vi "Process Collision.vi"(11 "Ball-Edge in":refnum<class "Ball-Edge.lvclass">) -> (3 "Ball-Edge out":refnum<class "Ball-Edge.lvclass">)   [LabVIEW 2021, in "Ball-Edge.lvclass"]
doc: "MIT Licence\nCopyright (c) 2024 David Grollier"
uses:
  Ball-Edge.lvclass
  C:/Users/David/Documents/GameSoccerSpace/Source/Collision/Collision.lvclass
  Collision type.ctl
  Game Componants/Game Board Component/Fixed/Board/Rectangle/Rectangle.lvclass
  Collision.lvclass/Collision.ctl
  Game Componants/Game Board Component/Movable/Movable.lvclass/Movable.ctl
  Game Componants/Game Board Component/Fixed/Board/Rectangle/Rectangle.lvclass/Rectangle.ctl
  Ball-Edge.lvclass/Ball-Edge.ctl
  Game Componants/Game Board Component/Movable/Movable.lvclass
  C:/Users/David/Documents/GameSoccerSpace/Source/Game Componants/Game Board Component/Game Board Component.lvclass
  Type Def/Coordinates.ctl
  Collision.lvclass
panel:
  out "sqrt(x)":dbl
  out "test type":T1
  out "test collision":bool
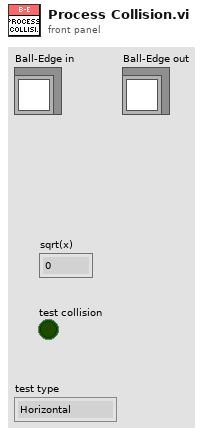
[diagram p1: front panel]
types:
  T1 = typedef "Ball-Edge.lvclass/Collision type.ctl" = enum16{"Horizontal", "Vertical", "Corner"}
  T2 = typedef "Coordinates.ctl" = cluster{"x":dbl, "y":dbl}
  T3 = cluster{"left":i16, "top":i16, "right":i16, "bottom":i16}
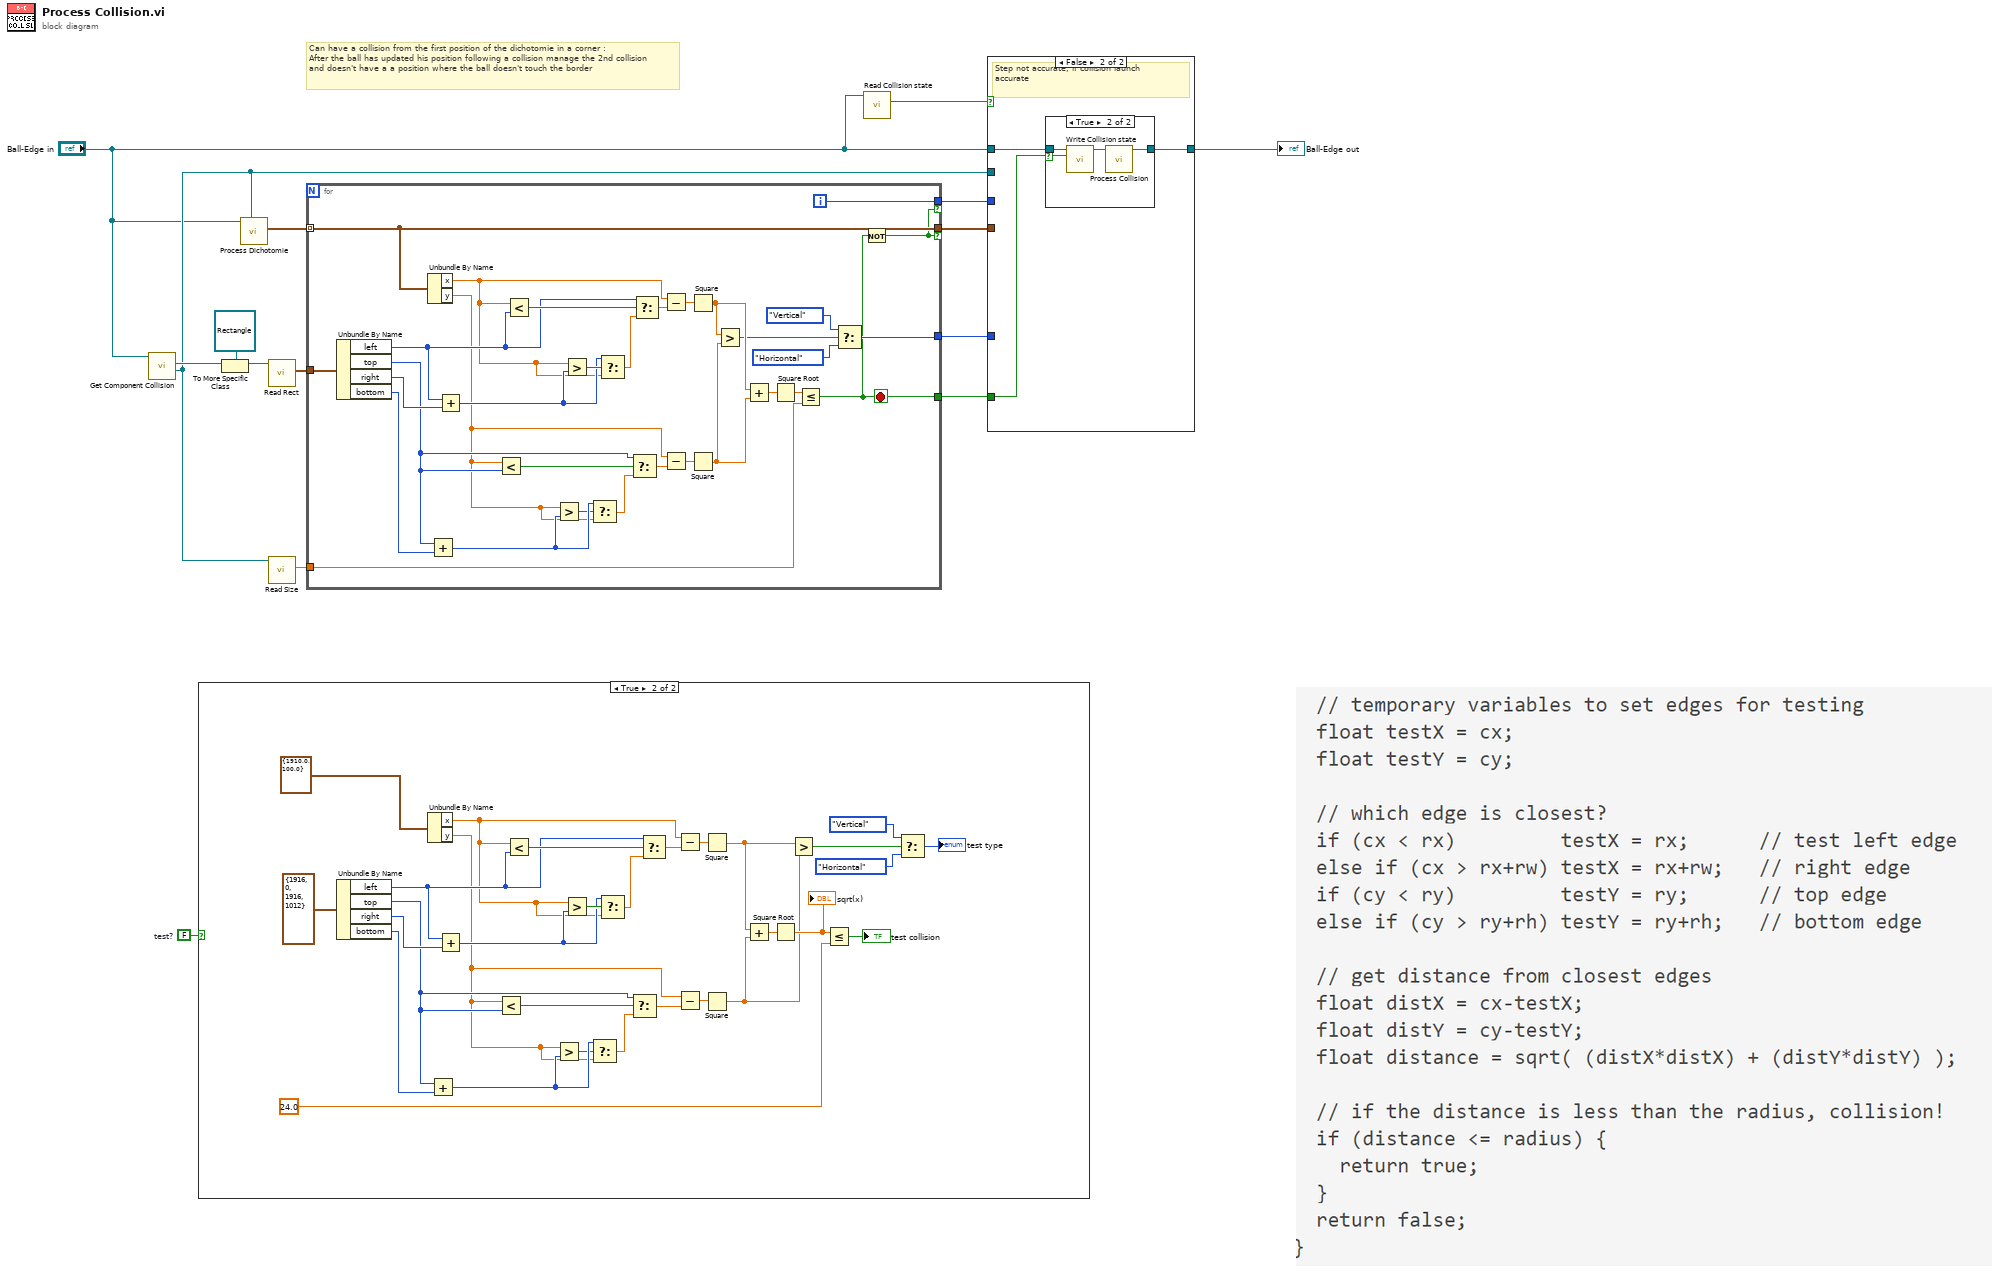
[diagram p0: block diagram]
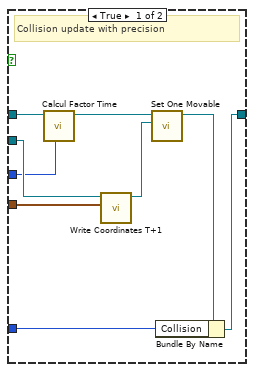
[diagram p2: hidden frame]
diagram:
  w8 = FALSE  # test?
  # "Can have a collision from the first position of the dichotomie in a corner :\nAfter the ball has updated his position following a collision manage the 2nd collision and doesn't have a a position where the ball doesn't touch the border"
  n1 = call "Get Component Collision.vi"("Collision in"="Ball-Edge in") -> ("Movable out"=w6:refnum<class "Movable.lvclass">, "GB Component out"=w13:refnum<class "Game Board Component.lvclass">)  [unwired: 9 in]
  n2 = case shown="True" w8 {
    frame False {
    }
    frame True {
      n3 = Unbundle By Name(T3 {"left"=1916, "top"=0, "right"=1916, "bottom"=1012} ("rect")) -> ("left"=w41:i16, "top"=w32:i16, "right"=w40:i16, "bottom"=w31:i16)
      n4 = Unbundle By Name(T2 {"x"=1910.0, "y"=100.0} ("Coordinates with dichotomie[]")) -> ("x"=w30:dbl, "y"=w28:dbl)
      n5 = Add(x=w32, y=w31) -> (x+y=w35:i16)
      n6 = Add(x=w41, y=w40) -> (x+y=w38:i16)
      n7 = Less?(x=w28, y=w32) -> (x < y?=w33:bool)
      n8 = Less?(x=w30, y=w41) -> (x < y?=w42:bool)
      n9 = Greater?(x=w28, y=w35) -> (0:w34:bool)
      n10 = Greater?(x=w30, y=w38) -> (0:w39:bool)
      n11 = Select(t=w35, s=w34, f=w28) -> (s? t:f=w36:dbl)
      n12 = Select(t=w38, s=w39, f=w30) -> (s? t:f=w37:dbl)
      n13 = Select(t=w32, s=w33, f=w36) -> (s? t:f=w27:dbl)
      n14 = Select(t=w41, s=w42, f=w37) -> (s? t:f=w29:dbl)
      n15 = Subtract(x=w30, y=w29) -> (x-y=w26:dbl)
      n16 = Subtract(x=w28, y=w27) -> (x-y=w25:dbl)
      n17 = Square(x=w26) -> (x^2=w22:dbl)
      n18 = Square(x=w25) -> (x^2=w21:dbl)
      n19 = Add(x=w22, y=w21) -> (x+y=w24:dbl)
      n20 = Square Root(x=w24) -> (sqrt(x)=w23:dbl)
      "sqrt(x)" <- w23
      n21 = Greater?(x=w22, y=w21) -> (0:w20:bool)
      n22 = Less Or Equal?(x=w23, y=24.0 ("Size")) -> (x <= y?=→"test collision":bool)
      n23 = Select(t=Collision_type."Vertical", s=w20, f=Collision_type."Horizontal") -> (s? t:f=→"test type":T1)
    }
  }
  n24 = To More Specific Class(target class=refnum<class "Rectangle.lvclass"> refnum ("Rectangle in"), reference=w13) -> (specific class reference=w12:refnum<class "Rectangle.lvclass">)  [unwired: 1 in, 1 out]
  n25 = call "Process Dichotomie.vi"("Movable in"=w6, "Collision in"="Ball-Edge in") -> ("Coordinates with dichotomie[] out"=w7:T2[])  [unwired: 8 in, 1 out]
  n26 = call "Read Rect.vi"("Rectangle in"=w12) -> ("rect"=w11:T3)  [unwired: 10 in]
  n27 = call "Read Size.vi"("Movable in"=w6) -> ("Size"=w15:dbl)  [unwired: 10 in]
  n28 = for {
    tunnel: [w48] -> w3
    tunnel: [w52] -> w10
    tunnel: w15 -> [w51]
    tunnel: w11 -> [w50]
    tunnel: w7 -> [w49] mode=indexing
    tunnel: [w46] -> w1 if=w47
    tunnel: [w49] -> w9 if=w47
    i -> [w46]
    stop <- w48 stop-if-true
    n29 = Unbundle By Name(w50) -> ("left"=w76:i16, "top"=w67:i16, "right"=w75:i16, "bottom"=w66:i16)
    n30 = Unbundle By Name(w49) -> ("x"=w65:dbl, "y"=w63:dbl)
    n31 = Add(x=w67, y=w66) -> (x+y=w70:i16)
    n32 = Add(x=w76, y=w75) -> (x+y=w73:i16)
    n33 = Less?(x=w63, y=w67) -> (x < y?=w68:bool)
    n34 = Less?(x=w65, y=w76) -> (x < y?=w77:bool)
    n35 = Greater?(x=w63, y=w70) -> (0:w69:bool)
    n36 = Greater?(x=w65, y=w73) -> (0:w74:bool)
    n37 = Select(t=w70, s=w69, f=w63) -> (s? t:f=w71:dbl)
    n38 = Select(t=w73, s=w74, f=w65) -> (s? t:f=w72:dbl)
    n39 = Select(t=w67, s=w68, f=w71) -> (s? t:f=w62:dbl)
    n40 = Select(t=w76, s=w77, f=w72) -> (s? t:f=w64:dbl)
    n41 = Subtract(x=w65, y=w64) -> (x-y=w61:dbl)
    n42 = Subtract(x=w63, y=w62) -> (x-y=w60:dbl)
    n43 = Square(x=w61) -> (x^2=w57:dbl)
    n44 = Square(x=w60) -> (x^2=w56:dbl)
    n45 = Greater?(x=w57, y=w56) -> (0:w55:bool)
    n46 = Add(x=w57, y=w56) -> (x+y=w59:dbl)
    n47 = Square Root(x=w59) -> (sqrt(x)=w58:dbl)
    n48 = Less Or Equal?(x=w58, y=w51) -> (x <= y?=w48:bool)
    n49 = Select(t=Collision_type."Vertical", s=w55, f=Collision_type."Horizontal") -> (s? t:f=w52:T1)
    n50 = Not(x=w48) -> (.not. x?=w47:bool)
  }
  n51 = call "Read Collision state.vi"("Collision in"="Ball-Edge in") -> ("Collision state"=w4:bool)  [unwired: 10 in]
  n52 = case shown="False" w4 {
    tunnel: w10 -> [w86 _]
    tunnel: [w85 w88] -> w2
    tunnel: w1 -> [w78 _]
    tunnel: w9 -> [w84 _]
    tunnel: w6 -> [w81 _]
    tunnel: "Ball-Edge in" -> [w80 w89]
    tunnel: w3 -> [_ w87]
    frame True {
      # "Collision update with precision"
      n53 = call "Calcul Factor Time.vi"("Accurate Iteration in"=w78, "Collision in"=w80) -> ("Collision out"=w79:refnum<class "Ball-Edge.lvclass">)  [unwired: 9 in]
      n54 = call "Write Coordinates T+1.vi"("Coordinates"=w84, "Movable in"=w81) -> ("Movable out"=w83:refnum<class "Movable.lvclass">)  [unwired: 9 in]
      n55 = call "Set One Movable.vi"("Movable in"=w83, "Collision in"=w79) -> ("Collision out"=w82:refnum<class "Ball-Edge.lvclass">)  [unwired: 9 in]
      n56 = Bundle By Name(cluster=w82, "Collision"=w86) -> (w85:refnum<class "Ball-Edge.lvclass">)
    }
    frame False {
      # "Step not accurate, if collision launch accurate"
      n57 = case shown="True" w87 {
        selector: w87 -> [_ w91]
        tunnel: w89 -> [w90 w93]
        tunnel: [w90 w92] -> w88
        frame False {
        }
        frame True {
          n58 = call "Write Collision state.vi"("Collision state"=w91, "Collision in"=w93) -> ("Collision out"=w94:refnum<class "Ball-Edge.lvclass">)  [unwired: 9 in]
          n59 = call-dynamic "Process Collision.vi"("Ball-Edge in"=w94) -> ("Ball-Edge out"=w92:refnum<class "Ball-Edge.lvclass">)  [unwired: 10 in]
        }
      }
    }
  }
  "Ball-Edge out" <- w2
